vi "Is_this_a_raw_data_file.vi"(0 "character string":string) -> (2 "Raw Dat File?":bool)   [LabVIEW 2010]
panel:
  out "Array":bool[](array[boolean])
  out "Output Array":string[](array[string])
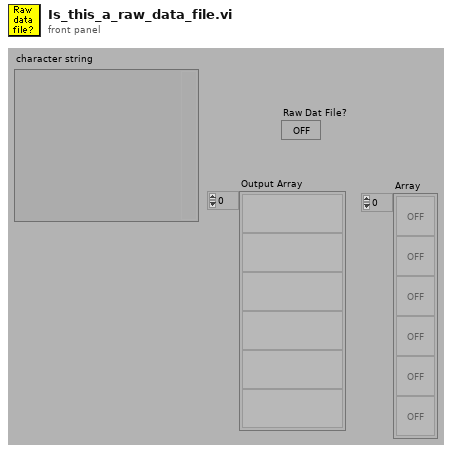
[diagram p1: front panel]
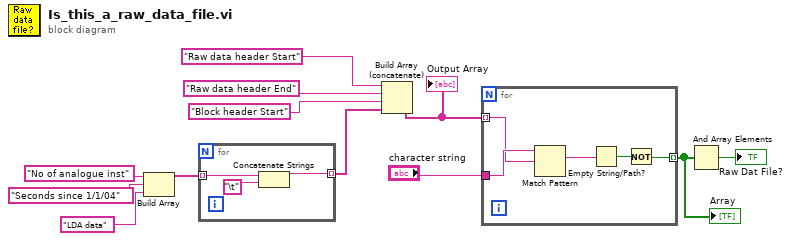
[diagram p0: block diagram]
diagram:
  n1 = Build Array("No of analogue inst", "Seconds since 1/1/04", "LDA data" ("Label for characters")) -> (w5:string[])
  n2 = for {
    tunnel: [w14] -> w12 mode=indexing
    tunnel: w5 -> [w13] mode=indexing
    n3 = Concatenate Strings(w13, "\t") -> (w14:string)
  }
  n4 = Build Array (concatenate)("Raw data header Start", "Raw data header End", "Block header Start", w12) -> (w10:string[])
  "Output Array" <- w10
  n5 = for {
    tunnel: "character string" -> [w20]
    tunnel: w10 -> [w19] mode=indexing
    tunnel: [w16] -> w9 mode=indexing
    n6 = Match Pattern(string=w20, regular expression=w19) -> (match substring=w18:string)  [unwired: 4 out]
    n7 = Empty String/Path?(string/path=w18) -> (empty?=w17:bool)
    n8 = Not(x=w17) -> (.not. x?=w16:bool)
  }
  "Array" <- w9
  n9 = And Array Elements(Boolean array=w9) -> (logical AND=→"Raw Dat File?":bool)
